vi "RootLocusSF.vi"() -> ()   [LabVIEW 2021]
uses:
  <vilib>/addons/Control Design/_Model Construction/Data Typedefs.llb/CD Variables.ctl
  <vilib>/addons/Control Design/_Model Construction/Data Typedefs.llb/CD Time Info.ctl
  <vilib>/Analysis/baseanly.llb/Real A x B.vi
  <vilib>/addons/Control Design/_Model Construction/Model Creation.llb/Model Creation SubVI/cd_Create State Space Model.vi
  <vilib>/Analysis/Matrix/Numeric/Subtract/Subtract - RM,RM.vi
  <vilib>/addons/Control Design/_Model Conversions/Model Type.llb/Model Conversion SubVI/cd_Convert State-Space to Zero-Pole-Gain Model.vi
  <vilib>/addons/Control Design/_Utility/Model Viewer.llb/Model Viewer SubVI/cd_Draw Zero-Pole-Gain Equation (ZPK).vi
  <vilib>/addons/Control Design/_Dynamic Analysis/Dynamic Analysis.llb/Dynamic Analysis subVI/cd_Root Locus (State-Space).vi
  <vilib>/addons/Control Design/_Utility/Model Viewer.llb/Model Viewer SubVI/cd_Draw State-Space Equation (SS).vi
  <vilib>/addons/Control Design/_Dynamic Analysis/Dynamic Analysis.llb/Dynamic Analysis subVI/cd_Poles (State-Space).vi
  <vilib>/addons/Control Design/_Time Response Analysis/Time Response.llb/Time Response subVI/cd_Initial Response (State-Space).vi
  <vilib>/addons/Control Design/_Model Construction/NI_LinSys_Model Creation.lvlib
  <vilib>/addons/Control Design/_Utility/NI_CD_Model Viewer.lvlib
  <vilib>/addons/Control Design/_Dynamic Analysis/NI_CD_Dynamic Analysis.lvlib
  <vilib>/addons/Control Design/_State-Space Analysis/NI_CD_State-Space Analysis.lvlib
  <vilib>/addons/Control Design/_Model Conversions/NI_CD_Model Type.lvlib
  <vilib>/addons/Control Design/_State Feedback Control/NI_CD_State Feedback Control.lvlib
  <vilib>/Analysis/NI_AALBase.lvlib
  <vilib>/Analysis/Matrix/NI_Matrix.lvlib
  <vilib>/addons/Control Design/_Time Response Analysis/NI_CD_Time Response.lvlib
  <vilib>/addons/Control Design/_Model Construction/NI_LinSys_Data Typedefs.lvlib
panel:
  out "Zero Pole Equation 2":picture
  out "1/J (B(2,1)":dbl
  out "L":dbl
  out "-b/J (A2,2)":dbl
  out "Original VS Full-State Feedback":cluster{"time":dbl[], dbl[]}[](graph)=[{"time"=[0.0, 0.1, 0.2, 0.30000000000000004, 0.4, 0.5, 0.6000000000000001, 0.7000000000000001, 0.8, 0.9, 1.0, 1.1, 1.2000000000000002, 1.3, 1.4000000000000001, 1.5, 1.6, 1.7000000000000002, 1.8, 1.9000000000000001, 2.0, 2.1, 2.2, 2.3000000000000003, 2.4000000000000004, 2.5, 2.6, 2.7, 2.8000000000000003, 2.9000000000000004, 3.0, 3.1, 3.2, 3.3000000000000003, 3.4000000000000004, 3.5, 3.6, 3.7, 3.8000000000000003, 3.9000000000000004, 4.0, 4.1000000000000005, 4.2, 4.3, 4.4, 4.5, 4.6000000000000005, 4.7, 4.800000000000001, 4.9, 5.0, 5.1000000000000005, 5.2, 5.300000000000001, 5.4, 5.5, 5.6000000000000005, 5.7, 5.800000000000001, 5.9, 6.0, 6.1000000000000005, 6.2, 6.300000000000001, 6.4, 6.5, 6.6000000000000005, 6.7, 6.800000000000001, 6.9, 7.0, 7.1000000000000005, 7.2, 7.300000000000001, 7.4, 7.5, 7.6000000000000005, 7.7, 7.800000000000001, 7.9, 8.0, 8.1, 8.200000000000001, 8.3, 8.4, 8.5, 8.6, 8.700000000000001, 8.8, 8.9, 9.0, 9.1, 9.200000000000001, 9.3, 9.4, 9.5, 9.600000000000001, 9.700000000000001, 9.8, 9.9, 10.0, 10.100000000000001, 10.200000000000001, 10.3, 10.4, 10.5, 10.600000000000001, 10.700000000000001, 10.8, 10.9, 11.0, 11.100000000000001, 11.200000000000001, 11.3, 11.4, 11.5, 11.600000000000001, 11.700000000000001, 11.8, 11.9, 12.0, 12.100000000000001, 12.200000000000001, 12.3, 12.4, 12.5, 12.600000000000001, 12.700000000000001, 12.8, 12.9, 13.0, 13.100000000000001, 13.200000000000001, 13.3, 13.4, 13.5, 13.600000000000001, 13.700000000000001, 13.8, 13.9, 14.0, 14.100000000000001, 14.200000000000001, 14.3, 14.4, 14.5, 14.600000000000001, 14.700000000000001, 14.8, 14.9, 15.0, 15.100000000000001, 15.200000000000001, 15.3, 15.4, 15.5, 15.600000000000001, 15.700000000000001, 15.8, 15.9, 16.0, 16.1, 16.2, 16.3, 16.400000000000002, 16.5, 16.6, 16.7, 16.8, 16.900000000000002, 17.0, 17.1, 17.2, 17.3, 17.400000000000002, 17.5, 17.6, 17.7, 17.8, 17.900000000000002, 18.0, 18.1, 18.2, 18.3, 18.400000000000002, 18.5, 18.6, 18.7, 18.8, 18.900000000000002, 19.0, 19.1, 19.200000000000003, 19.3, 19.400000000000002, 19.5, 19.6, 19.700000000000003, 19.8, 19.900000000000002, 20.0], [0.0, 0.0, 0.0, 0.0, 0.0, 0.0, 0.0, 0.0, 0.0, 0.0, 0.0, 0.0, 0.0, 0.0, 0.0, 0.0, 0.0, 0.0, 0.0, 0.0, 0.0, 0.0, 0.0, 0.0, 0.0, 0.0, 0.0, 0.0, 0.0, 0.0, 0.0, 0.0, 0.0, 0.0, 0.0, 0.0, 0.0, 0.0, 0.0, 0.0, 0.0, 0.0, 0.0, 0.0, 0.0, 0.0, 0.0, 0.0, 0.0, 0.0, 0.0, 0.0, 0.0, 0.0, 0.0, 0.0, 0.0, 0.0, 0.0, 0.0, 0.0, 0.0, 0.0, 0.0, 0.0, 0.0, 0.0, 0.0, 0.0, 0.0, 0.0, 0.0, 0.0, 0.0, 0.0, 0.0, 0.0, 0.0, 0.0, 0.0, 0.0, 0.0, 0.0, 0.0, 0.0, 0.0, 0.0, 0.0, 0.0, 0.0, 0.0, 0.0, 0.0, 0.0, 0.0, 0.0, 0.0, 0.0, 0.0, 0.0, 0.0, 0.0, 0.0, 0.0, 0.0, 0.0, 0.0, 0.0, 0.0, 0.0, 0.0, 0.0, 0.0, 0.0, 0.0, 0.0, 0.0, 0.0, 0.0, 0.0, 0.0, 0.0, 0.0, 0.0, 0.0, 0.0, 0.0, 0.0, 0.0, 0.0, 0.0, 0.0, 0.0, 0.0, 0.0, 0.0, 0.0, 0.0, 0.0, 0.0, 0.0, 0.0, 0.0, 0.0, 0.0, 0.0, 0.0, 0.0, 0.0, 0.0, 0.0, 0.0, 0.0, 0.0, 0.0, 0.0, 0.0, 0.0, 0.0, 0.0, 0.0, 0.0, 0.0, 0.0, 0.0, 0.0, 0.0, 0.0, 0.0, 0.0, 0.0, 0.0, 0.0, 0.0, 0.0, 0.0, 0.0, 0.0, 0.0, 0.0, 0.0, 0.0, 0.0, 0.0, 0.0, 0.0, 0.0, 0.0, 0.0, 0.0, 0.0, 0.0, 0.0, 0.0, 0.0, 0.0, 0.0, 0.0, 0.0, 0.0, 0.0]}, {"time"=[0.0, 0.1, 0.2, 0.30000000000000004, 0.4, 0.5, 0.6000000000000001, 0.7000000000000001, 0.8, 0.9, 1.0, 1.1, 1.2000000000000002, 1.3, 1.4000000000000001, 1.5, 1.6, 1.7000000000000002, 1.8, 1.9000000000000001, 2.0, 2.1, 2.2, 2.3000000000000003, 2.4000000000000004, 2.5, 2.6, 2.7, 2.8000000000000003, 2.9000000000000004, 3.0, 3.1, 3.2, 3.3000000000000003, 3.4000000000000004, 3.5, 3.6, 3.7, 3.8000000000000003, 3.9000000000000004, 4.0, 4.1000000000000005, 4.2, 4.3, 4.4, 4.5, 4.6000000000000005, 4.7, 4.800000000000001, 4.9, 5.0, 5.1000000000000005, 5.2, 5.300000000000001, 5.4, 5.5, 5.6000000000000005, 5.7, 5.800000000000001, 5.9, 6.0, 6.1000000000000005, 6.2, 6.300000000000001, 6.4, 6.5, 6.6000000000000005, 6.7, 6.800000000000001, 6.9, 7.0, 7.1000000000000005, 7.2, 7.300000000000001, 7.4, 7.5, 7.6000000000000005, 7.7, 7.800000000000001, 7.9, 8.0, 8.1, 8.200000000000001, 8.3, 8.4, 8.5, 8.6, 8.700000000000001, 8.8, 8.9, 9.0, 9.1, 9.200000000000001, 9.3, 9.4, 9.5, 9.600000000000001, 9.700000000000001, 9.8, 9.9, 10.0, 10.100000000000001, 10.200000000000001, 10.3, 10.4, 10.5, 10.600000000000001, 10.700000000000001, 10.8, 10.9, 11.0, 11.100000000000001, 11.200000000000001, 11.3, 11.4, 11.5, 11.600000000000001, 11.700000000000001, 11.8, 11.9, 12.0, 12.100000000000001, 12.200000000000001, 12.3, 12.4, 12.5, 12.600000000000001, 12.700000000000001, 12.8, 12.9, 13.0, 13.100000000000001, 13.200000000000001, 13.3, 13.4, 13.5, 13.600000000000001, 13.700000000000001, 13.8, 13.9, 14.0, 14.100000000000001, 14.200000000000001, 14.3, 14.4, 14.5, 14.600000000000001, 14.700000000000001, 14.8, 14.9, 15.0, 15.100000000000001, 15.200000000000001, 15.3, 15.4, 15.5, 15.600000000000001, 15.700000000000001, 15.8, 15.9, 16.0, 16.1, 16.2, 16.3, 16.400000000000002, 16.5, 16.6, 16.7, 16.8, 16.900000000000002, 17.0, 17.1, 17.2, 17.3, 17.400000000000002, 17.5, 17.6, 17.7, 17.8, 17.900000000000002, 18.0, 18.1, 18.2, 18.3, 18.400000000000002, 18.5, 18.6, 18.7, 18.8, 18.900000000000002, 19.0, 19.1, 19.200000000000003, 19.3, 19.400000000000002, 19.5, 19.6, 19.700000000000003, 19.8, 19.900000000000002, 20.0], [0.0, 0.0, 0.0, 0.0, 0.0, 0.0, 0.0, 0.0, 0.0, 0.0, 0.0, 0.0, 0.0, 0.0, 0.0, 0.0, 0.0, 0.0, 0.0, 0.0, 0.0, 0.0, 0.0, 0.0, 0.0, 0.0, 0.0, 0.0, 0.0, 0.0, 0.0, 0.0, 0.0, 0.0, 0.0, 0.0, 0.0, 0.0, 0.0, 0.0, 0.0, 0.0, 0.0, 0.0, 0.0, 0.0, 0.0, 0.0, 0.0, 0.0, 0.0, 0.0, 0.0, 0.0, 0.0, 0.0, 0.0, 0.0, 0.0, 0.0, 0.0, 0.0, 0.0, 0.0, 0.0, 0.0, 0.0, 0.0, 0.0, 0.0, 0.0, 0.0, 0.0, 0.0, 0.0, 0.0, 0.0, 0.0, 0.0, 0.0, 0.0, 0.0, 0.0, 0.0, 0.0, 0.0, 0.0, 0.0, 0.0, 0.0, 0.0, 0.0, 0.0, 0.0, 0.0, 0.0, 0.0, 0.0, 0.0, 0.0, 0.0, 0.0, 0.0, 0.0, 0.0, 0.0, 0.0, 0.0, 0.0, 0.0, 0.0, 0.0, 0.0, 0.0, 0.0, 0.0, 0.0, 0.0, 0.0, 0.0, 0.0, 0.0, 0.0, 0.0, 0.0, 0.0, 0.0, 0.0, 0.0, 0.0, 0.0, 0.0, 0.0, 0.0, 0.0, 0.0, 0.0, 0.0, 0.0, 0.0, 0.0, 0.0, 0.0, 0.0, 0.0, 0.0, 0.0, 0.0, 0.0, 0.0, 0.0, 0.0, 0.0, 0.0, 0.0, 0.0, 0.0, 0.0, 0.0, 0.0, 0.0, 0.0, 0.0, 0.0, 0.0, 0.0, 0.0, 0.0, 0.0, 0.0, 0.0, 0.0, 0.0, 0.0, 0.0, 0.0, 0.0, 0.0, 0.0, 0.0, 0.0, 0.0, 0.0, 0.0, 0.0, 0.0, 0.0, 0.0, 0.0, 0.0, 0.0, 0.0, 0.0, 0.0, 0.0, 0.0, 0.0, 0.0, 0.0, 0.0, 0.0]}]
  in  "Initial Conditions":dbl[](array[numeric])=[0.0, 0.0] format="%.3f"
  in  "Time Range":T1={"t0"=0.0, "dt"=0.1, "tf"=20.0} {"dt" format="%#.6g"; "tf" format="%#.6g"; "t0" format="%#.6g"}
  out "Controlled Root Locus Graph":cluster{dbl[], dbl[]}[](graph)=[{[], []}, {[-2.2500000000000004, -2.2500000000000004], [2.329999999999999, -2.329999999999999]}, {[], []}, {[], []}, {array[413 elements], array[413 elements]}, {array[413 elements], array[413 elements]}]
  out "closed loop State Space Equations":picture
  in  "D":dbl[][](array[numeric])=[[0.0]] format="%#.5g"
  in  "C":dbl[][](array[numeric])=[[1.0, 0.0]] format="%#.5g"
  in  "B":dbl[][](array[numeric])=[[0.0], [15.0]] format="%#.5g"
  in  "A":dbl[][](array[numeric])=[[0.0, 1.0], [0.0, -0.3]] format="%#.5g"
  in  "System's Parameters":T2 {"Value" format="%.2f"}
  in  "Desired Poles":cdb[](array[numeric])=[-2.25+2.33i, -2.25-2.33i] format="%.2f"
  in  "Gain Type":u16(ring) items=["Controller Gain", "Observer Gain (Predictive)", "Observer Gain (Current)"]
  out "State-Feedback Gain":dbl[][](array[numeric])=[[0.6994266666666668, 0.2800000000000001]] format="%.2f"
  out "Controllability Matrix":dbl[][](array[numeric])=[[0.0, 15.0], [15.0, -4.5]] format="%.2f"
  out "Zero Pole Equation":picture
  out "Is Controllable?":bool=TRUE
  out "OL Poles":cdb[](array[numeric])=[-0.3+0.0i, 0.0+0.0i] format="%.3f"
  out "Original System RL":cluster{dbl[], dbl[]}[](graph)=[{[-0.15000000000000024, -0.15000000000000024], [3.8700775186034715, -3.8700775186034715]}, {[-0.3, 0.0], [0.0, 0.0]}, {[], []}, {[-0.15], [0.0]}, {array[538 elements], array[538 elements]}, {array[538 elements], array[538 elements]}]
  in  "Gain":dbl[](array[numeric])=[1.0] format="%.2f"
  out "Open Loop State Space Equations":picture
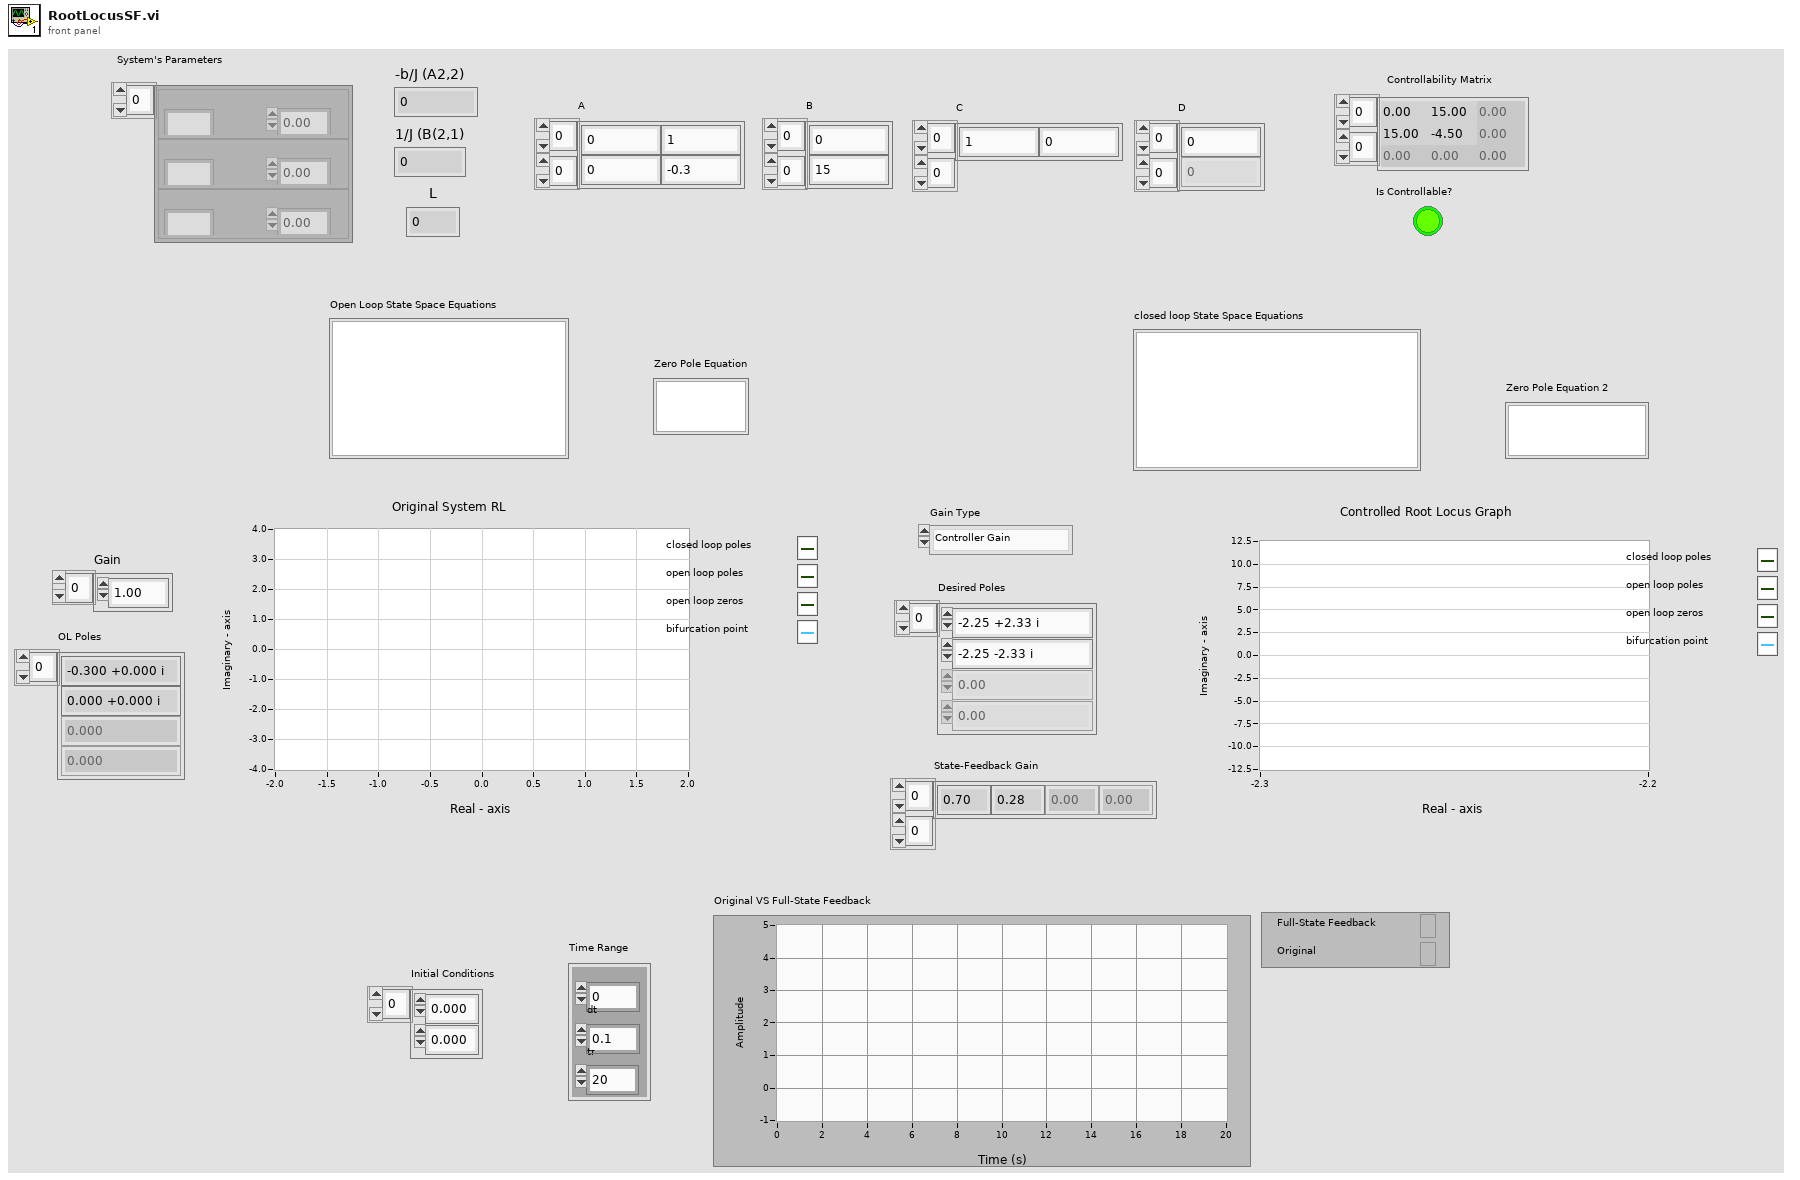
[diagram p1: front panel]
types:
  T1 = typedef "NI_LinSys_Data Typedefs.lvlib/CD Time Info.ctl" = cluster{"t0":dbl, "dt":dbl, "tf":dbl}
  T2 = typedef "NI_LinSys_Data Typedefs.lvlib/CD Variables.ctl" = cluster{"Name":string, " Value":dbl}[]
  T3 = typedef "NI_LinSys_Model Typedefs.lvlib/CD State Space Model (MIMO).ctl" = cluster{"properties":T4, "A":dbl[][], "B":dbl[][], "C":dbl[][], "D":dbl[][], "StateNames":string[], "Transport Delay":dbl[][]}
  T4 = typedef "NI_LinSys_Model Typedefs.lvlib/CD General Elements.ctl" = cluster{"Model name":string, "Input names":string[], "Output names":string[], "Input Delays":dbl[], "Output Delays":dbl[], "Sampling Time":dbl, "Notes":string}
  T5 = typedef "NI_LinSys_Model Typedefs.lvlib/CD Zero-Pole-Gain Model (MIMO).ctl" = cluster{"properties":T4, "zero-pole-gain(s)":T6[][]}
  T6 = typedef "NI_LinSys_Model Typedefs.lvlib/CD Zero-Pole-Gain Model (SISO).ctl" = cluster{"Gain":dbl, "Zeros":cdb[], "Poles":cdb[], "delay":dbl}
  T7 = typedef "NI_Matrix.lvlib/RealMatrix.ctl" = dbl[][]
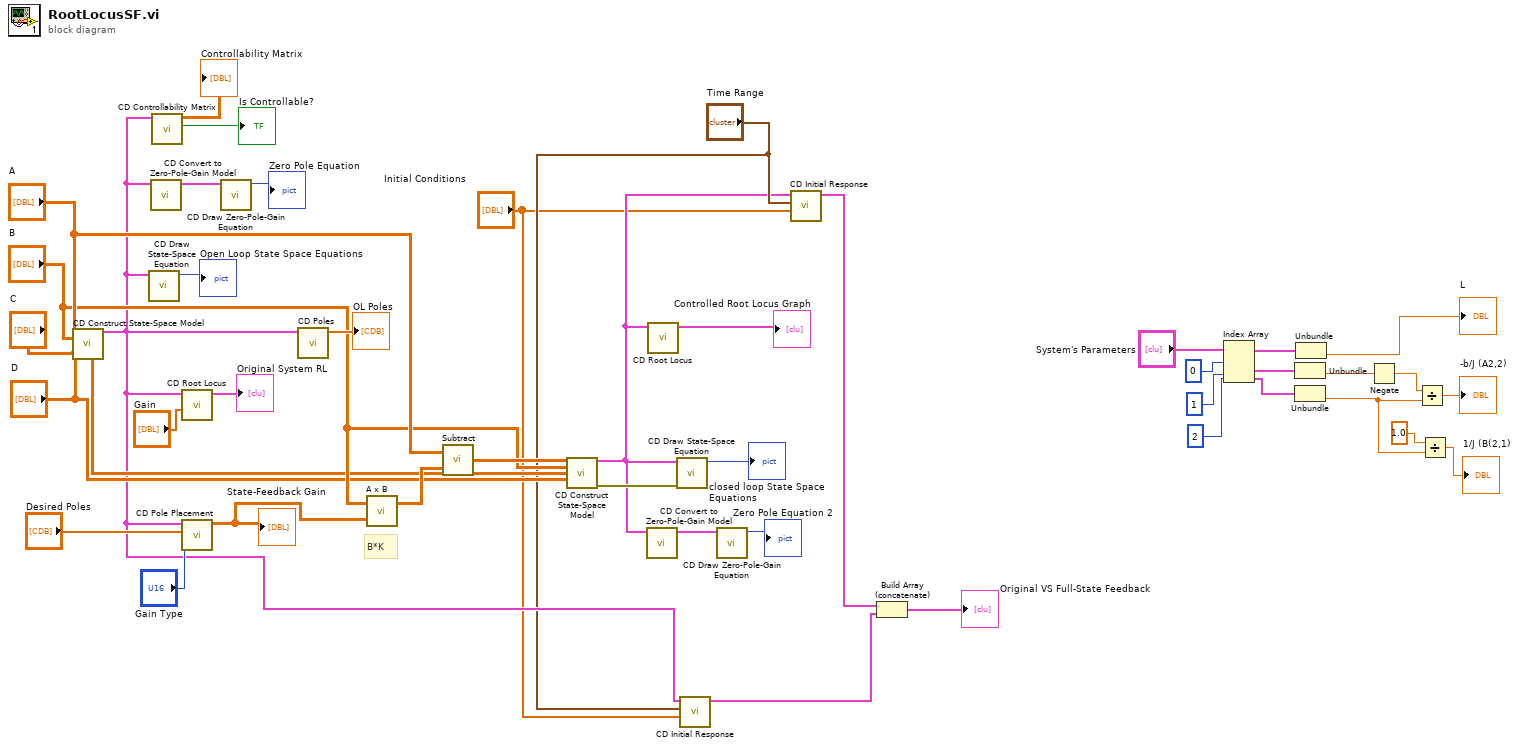
[diagram p0: block diagram]
diagram:
  # "B*K"
  n1 = call-poly <vilib>:"CD Construct State-Space Model.vi"("A"="A", "B"="B", "C"="C", "D"="D") -> ("State-Space Model"=w23:T3)  [unwired: 10 in, 1 out]
  n2 = call-poly <vilib>:"CD Draw State-Space Equation.vi"("State-Space Model"=w23) -> ("Equation"=→"Open Loop State Space Equations":picture)  [unwired: 8 in, 2 out]
  n3 = call-poly <vilib>:"CD Convert to Zero-Pole-Gain Model.vi"("State-Space Model"=w23) -> ("Zero-Pole-Gain Model"=w38:T5)  [unwired: 9 in, 1 out]
  n4 = call <vilib>:"CD Controllability Matrix.vi"("State-Space Model"=w23) -> ("Is Controllable?"=→"Is Controllable?":bool, "Controllability Matrix"=→"Controllability Matrix":dbl[][])  [unwired: 7 in, 2 out]
  n5 = call-poly <vilib>:"CD Root Locus.vi"("Gain"="Gain", "State-Space Model"=w23) -> ("Root Locus Graph"=→"Original System RL":cluster{dbl[], dbl[]}[])  [unwired: 6 in, 3 out]
  n6 = call <vilib>:"CD Pole Placement.vi"("Gain Type"="Gain Type", "Poles"="Desired Poles", "State-Space Model"=w23) -> ("Gain"=w31:dbl[][])  [unwired: 6 in, 2 out]
  "State-Feedback Gain" <- w31
  n7 = call-poly <vilib>:"CD Draw Zero-Pole-Gain Equation.vi"("Zero-Pole-Gain Model"=w38) -> ("Equation"=→"Zero Pole Equation":picture)  [unwired: 8 in, 2 out]
  n8 = call-poly <vilib>:"CD Poles.vi"("State-Space Model"=w23) -> ("Poles"=→"OL Poles":cdb[])  [unwired: 9 in, 1 out]
  n9 = call-poly <vilib>:"A x B.vi"("B"=w31, "A"="B") -> ("A x B"=w33:T7)  [unwired: 1 out]
  n10 = call-poly <vilib>:"Subtract.vi"("Real Matrix B"=w33, "Real Matrix A"="A") -> ("A - B"=w30:T7)
  n11 = call-poly <vilib>:"CD Construct State-Space Model.vi"("A"=w30, "B"="B", "C"="C", "D"="D") -> ("State-Space Model"=w2:T3, "error out"=w25:errorcluster)  [unwired: 10 in]
  n12 = call-poly <vilib>:"CD Convert to Zero-Pole-Gain Model.vi"("State-Space Model"=w2) -> ("Zero-Pole-Gain Model"=w4:T5)  [unwired: 9 in, 1 out]
  n13 = call-poly <vilib>:"CD Root Locus.vi"("State-Space Model"=w2) -> ("Root Locus Graph"=→"Controlled Root Locus Graph":cluster{dbl[], dbl[]}[])  [unwired: 7 in, 3 out]
  n14 = call-poly <vilib>:"CD Draw State-Space Equation.vi"("error in (no error)"=w25, "State-Space Model"=w2) -> ("Equation"=→"closed loop State Space Equations":picture)  [unwired: 7 in, 2 out]
  n15 = call-poly <vilib>:"CD Initial Response.vi"("Initial Conditions"="Initial Conditions", "Time Range"="Time Range", "State-Space Model"=w23) -> ("Initial Response Graph"=w21:cluster{"time":dbl[], dbl[]}[])  [unwired: 5 in, 3 out]
  n16 = call-poly <vilib>:"CD Draw Zero-Pole-Gain Equation.vi"("Zero-Pole-Gain Model"=w4) -> ("Equation"=→"Zero Pole Equation 2":picture)  [unwired: 8 in, 2 out]
  n17 = call-poly <vilib>:"CD Initial Response.vi"("Initial Conditions"="Initial Conditions", "Time Range"="Time Range", "State-Space Model"=w2) -> ("Initial Response Graph"=w20:cluster{"time":dbl[], dbl[]}[])  [unwired: 5 in, 3 out]
  n18 = Build Array (concatenate) "Build Array"(w20, w21) -> (→"Original VS Full-State Feedback":cluster{"time":dbl[], dbl[]}[])
  n19 = Index Array(array="System's Parameters", index #1=0 ("index"), index #2=1 ("index"), index #3=2 ("index")) -> (element #1=w14:cluster{"Name":string, " Value":dbl}, element #2=w13:cluster{"Name":string, " Value":dbl}, element #3=w12:cluster{"Name":string, " Value":dbl})
  n20 = Unbundle(w13) -> ("Value"=w11:dbl)  [unwired: 1 out]
  n21 = Unbundle(w12) -> ("Value"=w6:dbl)  [unwired: 1 out]
  n22 = Unbundle(w14) -> ("Value"=→"L":dbl)  [unwired: 1 out]
  n23 = Negate(x=w11) -> (-x=w10:dbl)
  n24 = Divide(x=w10, y=w6) -> (x/y=→"-b/J (A2,2)":dbl)
  n25 = Divide(x=1.0, y=w6) -> (x/y=→"1/J (B(2,1)":dbl)
